vi "testUnflattenAngularVelocityFromXML.vi"() -> ()   [LabVIEW 2012, in "UnitsAndXML.lvlib"]
uses:
  <userlib>/Common/UnitsAndXML/UnitsAndXML.lvlib
  <userlib>/Common/UnitsAndXML/FlattenItemWithUnitToXML/FlattenAngularVelocityToXML/AngularVelocityUnit.ctl
  <userlib>/Common/UnitsAndXML/UnflattenItemWithUnitFromXML/UnflattenAngularVelocityFromXML/typeMethods/unflattenAngularVelocityFromXML_Array.vi
  <userlib>/Common/UnitsAndXML/UnflattenItemWithUnitFromXML/UnflattenAngularVelocityFromXML/typeMethods/unflattenAngularVelocityFromXML_Scalar.vi
panel:
  out "error out":errorcluster
  out "angularVelocity":dbl[unit][](array[numeric])
  out "angularVelocity":dbl[unit]
  in  "angularVelocityUnitInXML":T1
  in  "xmlStringArray":string="<velocity>15</velocity>\r\n<velocity>30</velocity>\r\n<velocity>45</velocity>\r\n<velocity>60</velocity>"
  in  "xmlStringScalar":string="<velocity>15</velocity>"
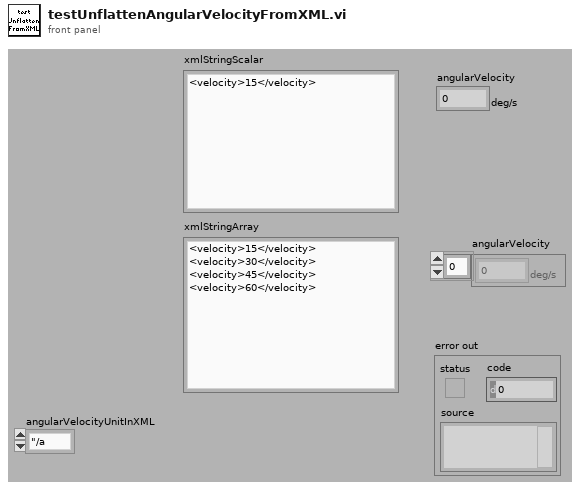
[diagram p1: front panel]
types:
  T1 = typedef "UnitsAndXML.lvlib/AngularVelocityUnit.ctl" = enum16{"\"/a", "deg/s", "\"/s"}
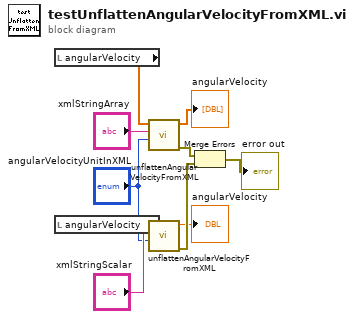
[diagram p0: block diagram]
diagram:
  n1 = local read "angularVelocity"() -> (w3:dbl[unit][])
  n2 = local read "angularVelocity"() -> (w10:dbl[unit])
  n3 = call-poly <userlib>:"unflattenAngularVelocityFromXML.vi"("angularVelocityUnitInXML"="angularVelocityUnitInXML", "xmlString"="xmlStringArray", "angularVelocityForType"=w3) -> ("error out"=w7:errorcluster, "angularVelocity"=→"angularVelocity":dbl[unit][])  [unwired: 7 in]
  n4 = call-poly <userlib>:"unflattenAngularVelocityFromXML.vi"("angularVelocityUnitInXML"="angularVelocityUnitInXML", "xmlString"="xmlStringScalar", "angularVelocityForType"=w10) -> ("error out"=w6:errorcluster, "angularVelocity"=→"angularVelocity":dbl[unit])  [unwired: 7 in]
  n5 = Merge Errors(w7, w6) -> (→"error out":errorcluster)
